vi "FPGAInterface.vi"(8 "error in (no error)":errorcluster, 11 "User Event in":refnum<class "User Event.lvclass">) -> (0 "error out":errorcluster)   [LabVIEW 2018]
uses:
  User Events/User Event.lvclass
  <vilib>/FPGAPlugInAG/cRIO-9039 (Sync)/niLvFpga_Open_cRIO-9039 (Sync).vi
  <vilib>/rvi/interface/common/dynamic/niFpgaDynamicAddResources.vi
  <vilib>/FPGAPlugInAG/Dynamic/niLvFpga_Abort_Dynamic.vi
  <vilib>/FPGAPlugInAG/Dynamic/niLvFpga_Reset_Dynamic.vi
  <vilib>/FPGAPlugInAG/Dynamic/niLvFpga_Run_Dynamic.vi
  <vilib>/Utility/error.llb/Error Cluster From Error Code.vi
  <vilib>/rvi/errors/niLvFpgaAdjustHostInterfaceError.vi
  <vilib>/FPGAPlugInAG/Dynamic/niLvFpga_Close_Dynamic.vi
  <vilib>/rvi/interface/nirviOpenFPGA/nirviOpenFPGA.xnode
  FPGA Bitfiles/M1M3SupportSimulator.lvbitx
  <vilib>/rvi/interface/nirviMethod/nirviMethod.xnode
  <vilib>/rvi/interface/nirviCloseFPGA/nirviCloseFPGA.xnode
  <vilib>/FPGAPlugInAG/Dynamic/niLvFpga_ReadFifo_Dynamic.vi
  <vilib>/rvi/errors/niLvFpgaMergeErrorWithErrorCode.vi
  <vilib>/FPGAPlugInAG/Dynamic/niLvFpga_WriteFifo_Dynamic.vi
panel:
  out "Data":u32[](array[numeric])
  in  "Stop Button":bool
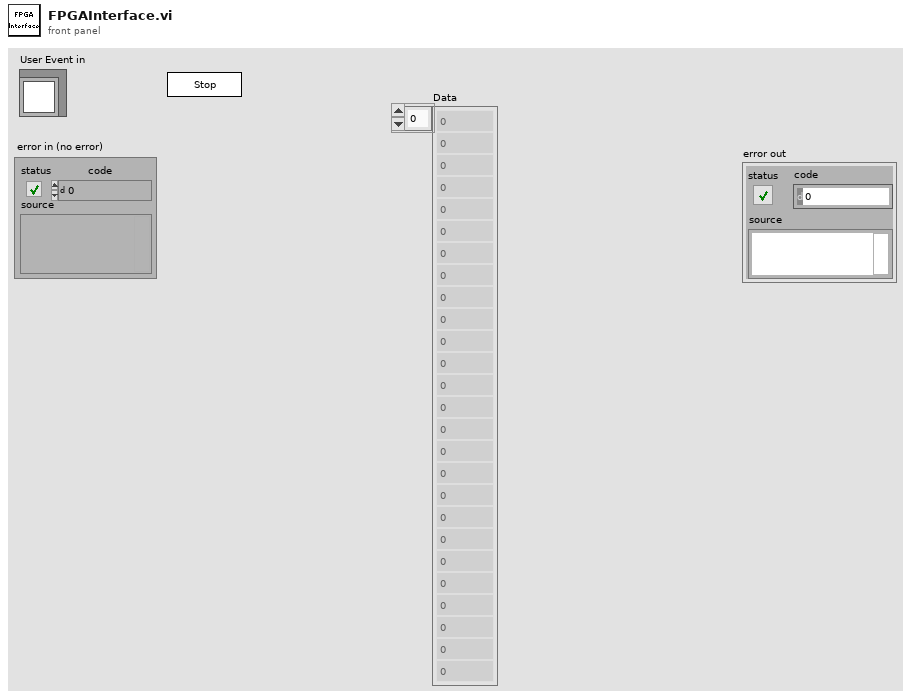
[diagram p1: front panel]
types:
  T1 = typedef "M1M3SupSimUserEvents.ctl" = cluster{"ILCResponse":refnum<user-event>, "StopUDPServer":refnum<user-event>}
  T2 = cluster{"Event Registration Refnum":refnum<event-registration>, "Event Registration Refnum":refnum<event-registration>}
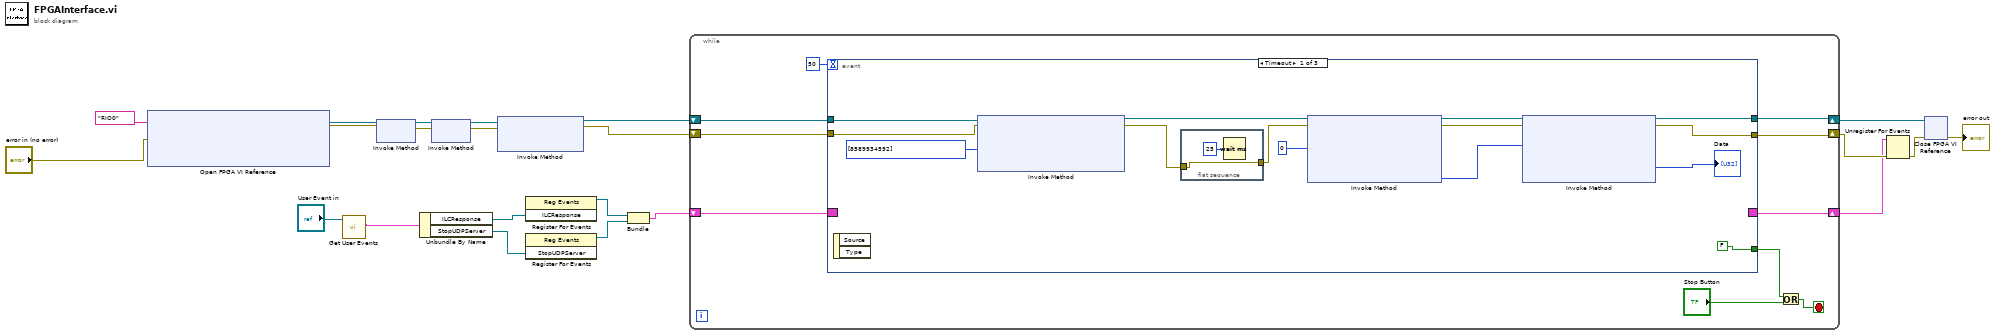
[diagram p0: block diagram]
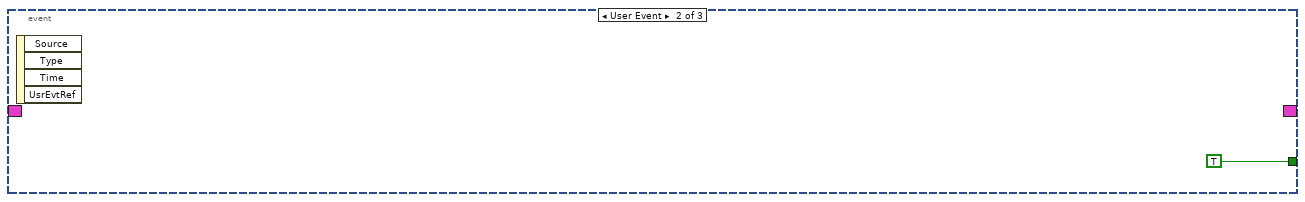
[diagram p2: hidden frame]
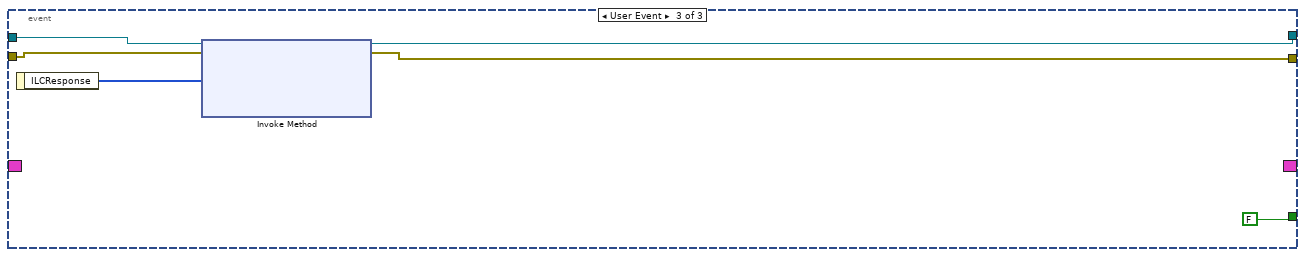
[diagram p3: hidden frame]
diagram:
  n1 = xnode "Open FPGA VI Reference"("error in"="error in (no error)", "resource name"=tag "RIO0") -> ("FPGA VI Reference Out"=w22:refnum<k20>, "error out"=w16:errorcluster)
  n2 = call "Get User Events.vi"("User Event in"="User Event in") -> ("User Events"=w1:T1)  [unwired: 8 in, 2 out]
  n3 = xnode "Invoke Method"("FPGA VI Reference In"=w22, "error in"=w16) -> ("FPGA VI Reference Out"=w21:refnum<k20>, "error out"=w15:errorcluster)
  n4 = Unbundle By Name(w1) -> ("ILCResponse"=w12:refnum<user-event>, "StopUDPServer"=w10:refnum<user-event>)
  n5 = xnode "Invoke Method"("FPGA VI Reference In"=w21, "error in"=w15) -> ("FPGA VI Reference Out"=w20:refnum<k20>, "error out"=w14:errorcluster)
  n6 = xnode "Invoke Method"("FPGA VI Reference In"=w20, "error in"=w14) -> ("FPGA VI Reference Out"=w17:refnum<k20>, "error out"=w11:errorcluster)  [unwired: 1 in]
  n7 = register-events(w12) -> (reference out=w9:refnum<event-registration>)  [unwired: 2 in, 1 out]
  n8 = register-events(w10) -> (reference out=w8:refnum<event-registration>)  [unwired: 2 in, 1 out]
  n9 = Bundle("Event Registration Refnum"=w9, "Event Registration Refnum"=w8) -> (w7:T2)  [unwired: 1 in]
  n10 = while {
    shift-right: [w30] -> w19
    shift-left: w17 -> [w31]
    shift-right: [w32] -> w3
    shift-left: w7 -> [w23]
    shift-right: [w27] -> w5
    shift-left: w11 -> [w28]
    stop <- w26 stop-if-true
    n11 = event shown="[0] Timeout" {
      selector: w23 -> [_ _ _]
      dyn-events: [_ _ _] -> w32
      timeout: 50 -> [_ _ _]
      tunnel: w31 -> [w46 _ w55]
      tunnel: [w38 _ w54] -> w30
      tunnel: w28 -> [w36 _ w53]
      tunnel: [w34 _ w52] -> w27
      tunnel: [FALSE TRUE FALSE] -> w24
      event Timeout {
        n12 = event-data() -> ()  [unwired: 1 in, 2 out]
        n13 = xnode "Invoke Method"("FPGA VI Reference In"=w46, "error in"=w36, "Data"=u64[] [8589934592]) -> ("FPGA VI Reference Out"=w41:refnum<k20>, "error out"=w43:errorcluster)  [unwired: 1 in, 1 out]
        n14 = flat-sequence {
          tunnel: [w48] -> w44
          tunnel: w43 -> [w48]
          frame #0 {
            n15 = Wait (ms)(milliseconds to wait=u32 25) -> ()  [unwired: 1 out]
          }
        }
        n16 = xnode "Invoke Method"("FPGA VI Reference In"=w41, "error in"=w44, "Number of Elements"=u32 0) -> ("FPGA VI Reference Out"=w40:refnum<k20>, "error out"=w35:errorcluster, "Elements Remaining"=w39:u32)  [unwired: 1 in, 1 out]
        n17 = xnode "Invoke Method"("FPGA VI Reference In"=w40, "error in"=w35, "Number of Elements"=w39) -> ("FPGA VI Reference Out"=w38:refnum<k20>, "error out"=w34:errorcluster, "Data"=→"Data":u32[])  [unwired: 1 in, 1 out]
      }
      event User Event {
        n18 = event-data() -> ()  [unwired: 1 in, 4 out]
      }
      event User Event {
        n19 = event-data() -> ("ILCResponse"=w50:u8[])  [unwired: 1 in]
        n20 = xnode "Invoke Method"("FPGA VI Reference In"=w55, "error in"=w53, "Data"=w50) -> ("FPGA VI Reference Out"=w54:refnum<k20>, "error out"=w52:errorcluster)  [unwired: 1 in, 1 out]
      }
    }
    n21 = Or(x=w24, y="Stop Button") -> (x .or. y?=w26:bool)
  }
  n22 = Unregister For Events(event registration refnum=w3, error in=w5) -> (error out=w6:errorcluster)
  n23 = xnode "Close FPGA VI Reference"("FPGA VI Reference In"=w19, "error in"=w6) -> ("error out"=→"error out":errorcluster)
